vi "Validate Project Path.vi"(0 "Project path in":path, 5 "LabVIEW Version":string, 11 "error in (no error)":errorcluster) -> (4 "Validated project path":path, 6 "New project?":bool, 8 "Warning":string, 15 "error out":errorcluster)   [LabVIEW 2021, in "Converter.lvlib"]
uses:
  Converter.lvlib
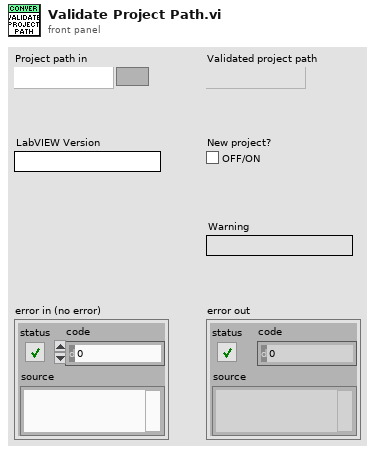
[diagram p1: front panel]
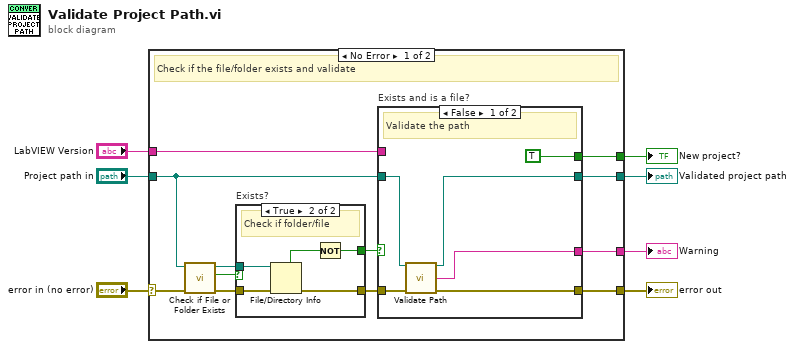
[diagram p0: block diagram]
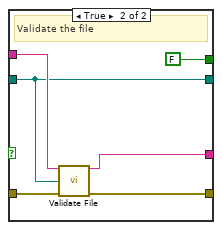
[diagram p2: hidden frame]
diagram:
  n1 = case shown="No Error" "error in (no error)" {
    selector: "error in (no error)" -> [w14 w38]
    tunnel: [w19 _] -> w7
    tunnel: [w18 w39] -> w6
    tunnel: "Project path in" -> [w11 w39]
    tunnel: [w17 w38] -> w4
    tunnel: [w16 _] -> w3
    tunnel: "LabVIEW Version" -> [w13 _]
    frame No Error {
      # "Check if the file/folder exists and validate"
      n2 = call <vilib>:"Check if File or Folder Exists.vi"("error in (no error)"=w14, "path"=w11) -> ("error out"=w12:errorcluster, "file or folder exists?"=w10:bool, "dup path"=w9:path)  [unwired: 7 in]
      n3 = case "Exists?" shown="True" w10 {
        tunnel: [w32 w37] -> w15
        tunnel: w12 -> [w32 w36]
        tunnel: w9 -> [_ w35]
        tunnel: [_ w34] -> w8
        frame False {
          # "Pass"
        }
        frame True {
          # "Check if folder/file"
          n4 = File/Directory Info(path=w35, error in=w36) -> (directory=w33:bool, error out=w37:errorcluster)  [unwired: 5 out]
          n5 = Not(x=w33) -> (.not. x?=w34:bool)
        }
      }
      n6 = case "Exists and is a file?" shown="False" w8 {
        tunnel: w15 -> [w25 w31]
        tunnel: w13 -> [_ w30]
        tunnel: w11 -> [w23 w27]
        tunnel: [w22 w28] -> w16
        tunnel: [w24 w29] -> w17
        tunnel: [w21 w27] -> w18
        tunnel: [TRUE ("New project?") FALSE ("New project?")] -> w19
        frame False {
          # "Validate the path"
          n7 = call "Validate Path.vi"("Input path"=w23, "error in (no error)"=w25) -> ("Validated path"=w21:path, "Warning"=w22:string, "error out"=w24:errorcluster)  [unwired: 11 in]
        }
        frame True {
          # "Validate the file"
          n8 = call "Validate File.vi"("LabVIEW version"=w30, "Project path"=w27, "error in (no error)"=w31) -> ("Warning"=w28:string, "error out"=w29:errorcluster)  [unwired: 11 in]
        }
      }
    }
    frame Error {
      # "Pass"
    }
  }
  "New project?" <- w7
  "Validated project path" <- w6
  "error out" <- w4
  "Warning" <- w3
